vi "Set Server State UE.vi"(10 "Server State UE":refnum<user-event>, 11 "Template Server in":refnum<class "OCV2.lvclass">) -> (3 "Template Server out":refnum<class "OCV2.lvclass">)   [LabVIEW 2019, in "OCV2.lvlib" / "OCV2.lvclass"]
uses:
  OCV2.lvclass
  typeDefs/Server State Data.ctl
  OCV2.lvclass/OCV2.ctl
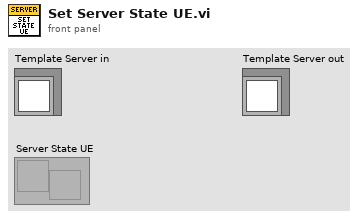
[diagram p1: front panel]
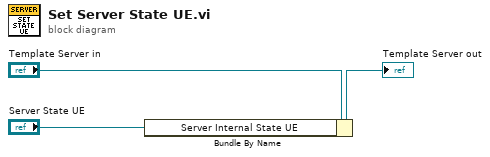
[diagram p0: block diagram]
diagram:
  n1 = Bundle By Name(cluster="Template Server in", "Server Internal State UE"="Server State UE") -> (→"Template Server out":refnum<class "OCV2.lvclass">)
